vi "Camera AE V1.0.vi"(6 ".NET (Reference)":refnum<k24>, 7 "Camera Control In":T1 {"Frame Rate (fps)" scale=0.0..10.0; "Exposure Time (ms)" scale=0.0..10.0; "Pixel Clock (MHz)" scale=0.0..10.0}, 8 "Camera ID":i32, 9 "Action":T2) -> (0 "Error Out":errorcluster, 1 "Camera Control Out":T1 {"Frame Rate (fps)" scale=0.0..10.0; "Exposure Time (ms)" scale=0.0..10.0; "Pixel Clock (MHz)" scale=0.0..10.0}, 2 "Reference Out":refnum<k24>, 3 "Array":u8[][](array[numeric]))   [LabVIEW 2014]
uses:
  Controls/Standard Action for Camera Control.ctl
  C:/Program Files (x86)/National Instruments/LabVIEW 2014/instr.lib/IDS/ueye.NET/uEyeDotNet.dll
  Program Files (x86)/National Instruments/LabVIEW 2014/instr.lib/IDS/ueye.NET/uEyeDotNet.dll
  Controls/Camera Control.ctl
panel:
  out "Bits/Pixel":i32=8
  out "Width":i32=8
  out "Height":i32=8
  out "Serial Number 1":string
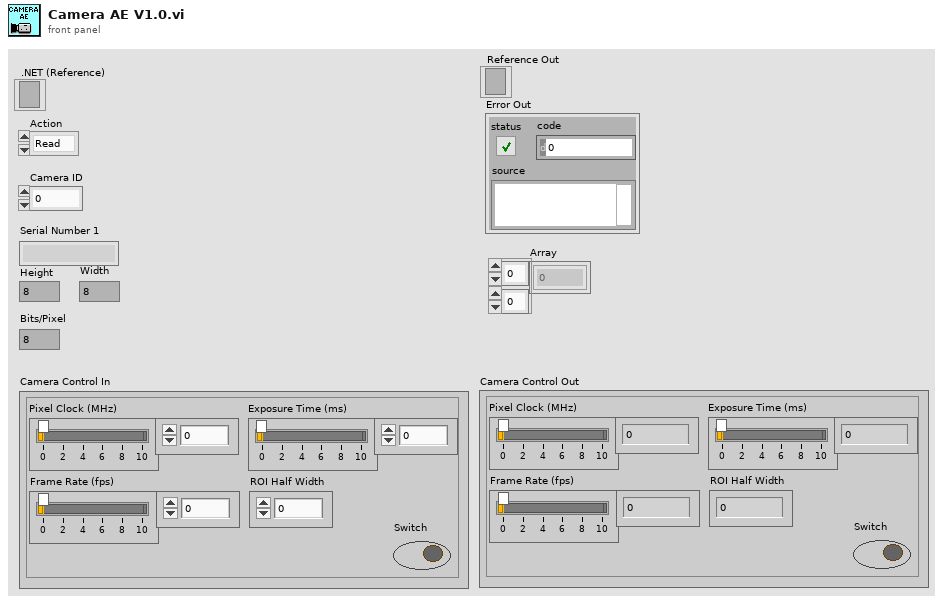
[diagram p1: front panel]
types:
  T1 = typedef "Camera Control.ctl" = cluster{"Pixel Clock (MHz)":i32, "Exposure Time (ms)":dbl, "Frame Rate (fps)":dbl, "ROI Half Width":i32, "Switch":bool}
  T2 = typedef "Standard Action for Camera Control.ctl" = enum16{"Read", "Setting", "Switch", "Initialization", "Exit"}
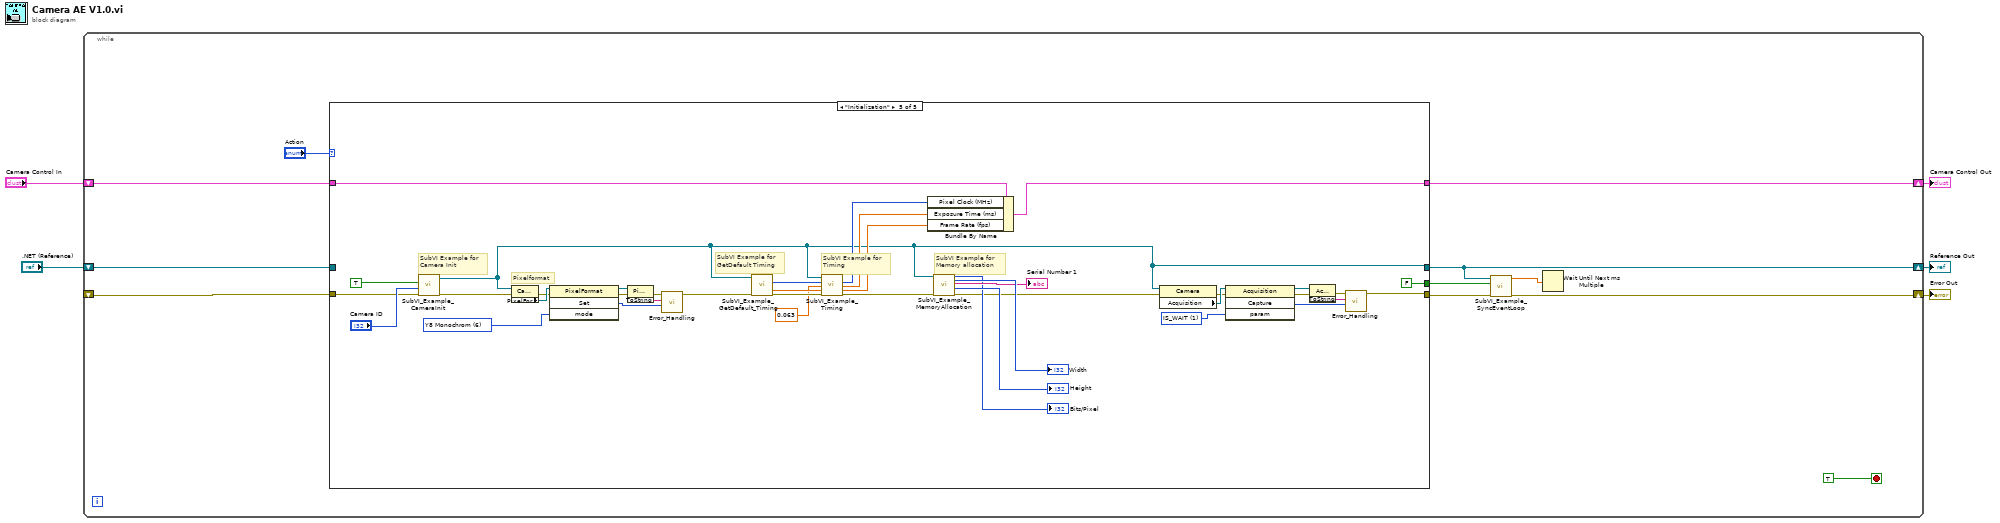
[diagram p0: block diagram]
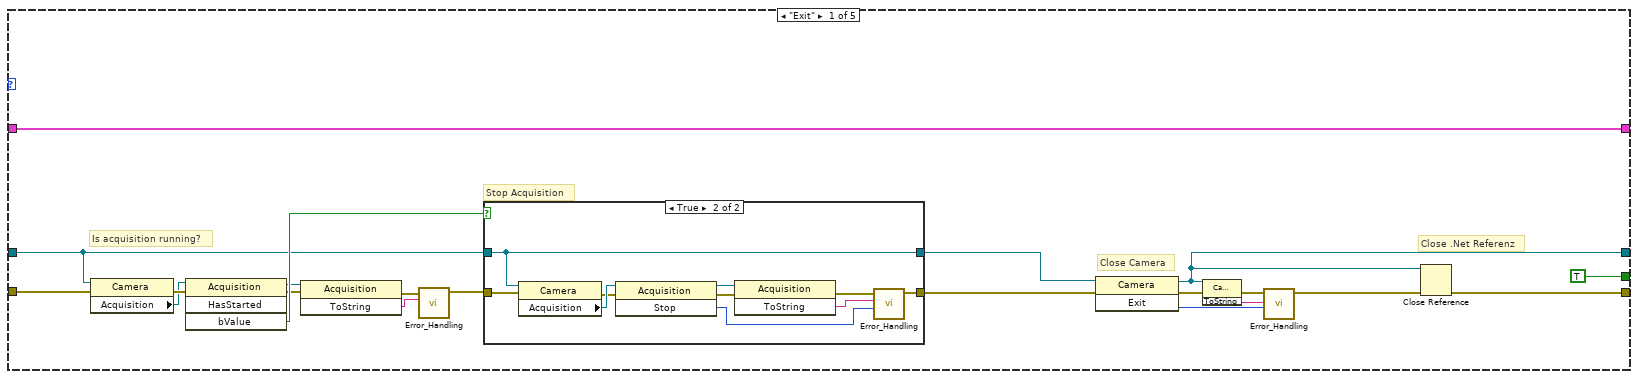
[diagram p2: hidden frame]
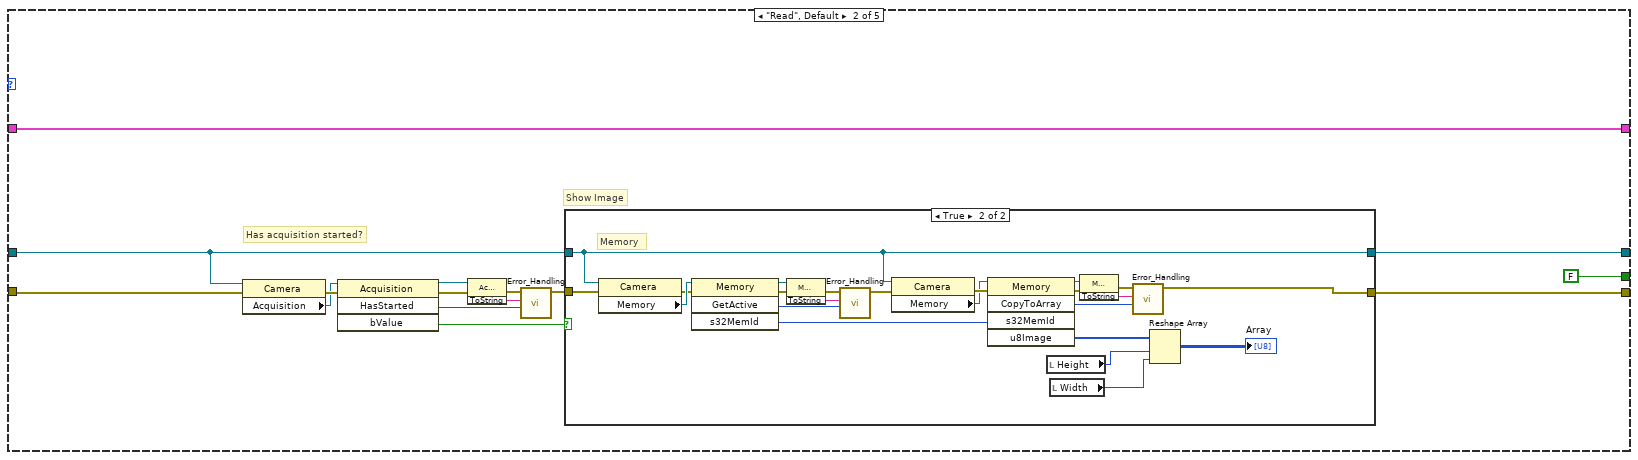
[diagram p4: hidden frame]
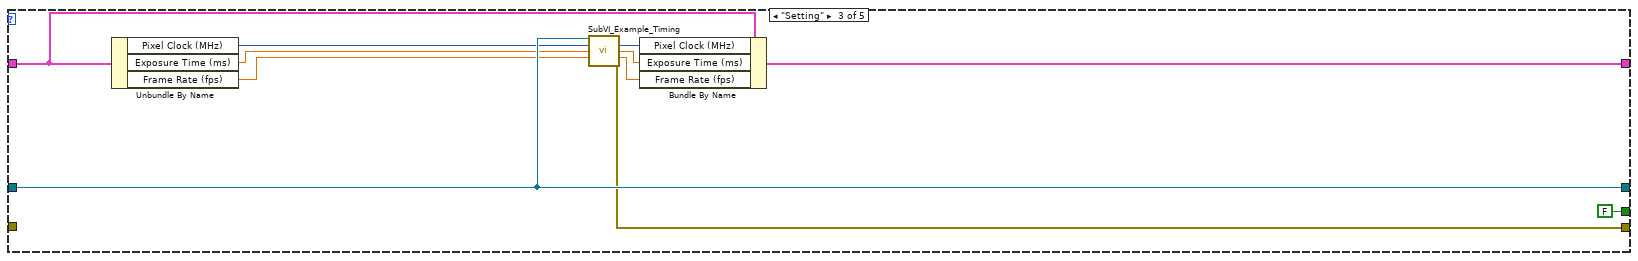
[diagram p6: hidden frame]
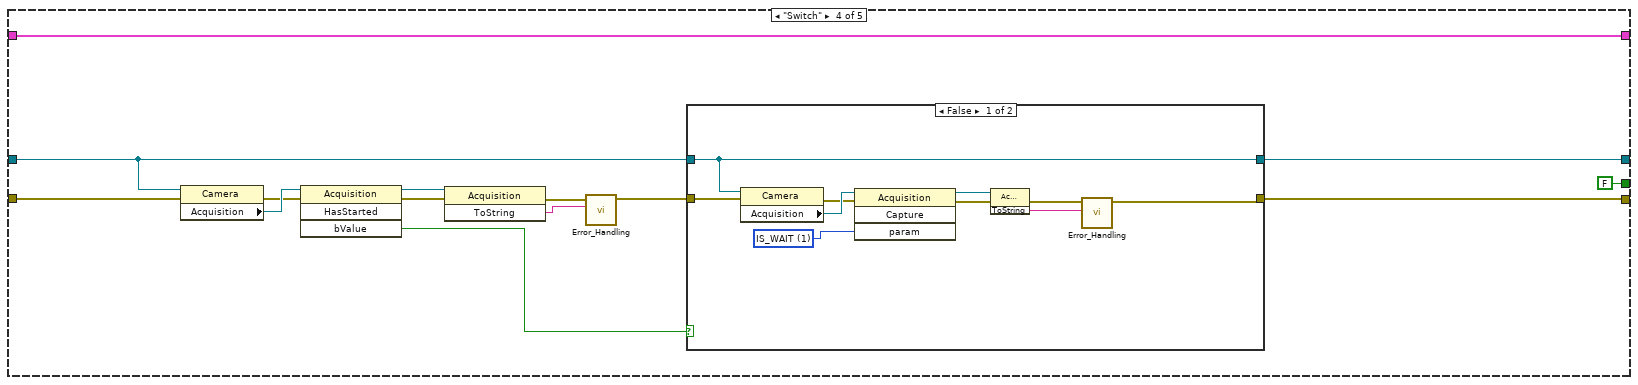
[diagram p7: hidden frame]
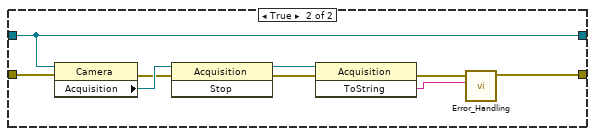
[diagram p8: hidden frame]
diagram:
  n1 = while {
    shift-right: [w12] -> w4
    shift-left: _ -> [w15]
    shift-right: [w13] -> w5
    shift-left: ".NET (Reference)" -> [w16]
    shift-right: [w7] -> w2
    shift-left: "Camera Control In" -> [w6]
    stop <- TRUE stop-if-true
    n2 = case shown="\"Initialization\"" "Action" {
      tunnel: w16 -> [w21 w53 w99 w101 _]
      tunnel: w15 -> [w22 w52 _ w114 w164]
      tunnel: [w31 w55 w99 w106 w136] -> w13
      tunnel: [w32 w54 w92 w103 w144] -> w14
      tunnel: [TRUE FALSE FALSE FALSE FALSE] -> w10
      tunnel: [w17 w50 w93 w111 w138] -> w7
      tunnel: w6 -> [w17 w50 w96 w111 w141]
      frame "Exit" {
        # "Close .Net Referenz"
        # "Is acquisition running?"
        # "Stop Acquisition"
        # "Close Camera"
        n3 = property class="Camera"(reference=w21, error in=w22) -> (error out=w30:errorcluster, "Acquisition"=w29:refnum<k24>)  [unwired: 1 out]
        n4 = invoke class="Acquisition" method="HasStarted"(reference=w29, error in=w30) -> (reference out=w23:refnum<k24>, error out=w26:errorcluster, "bValue"=w28:bool)  [unwired: 2 in, 1 out]
        n5 = invoke class="Acquisition" method="ToString"(reference=w23, error in=w26) -> (error out=w25:errorcluster, "ToString"=w24:string)  [unwired: 1 in, 1 out]
        n6 = call <instrlib>:"Error_Handling.vi"("Error String"=w24, "Error In"=w25) -> ("Error Out"=w27:errorcluster)  [unwired: 9 in]
        n7 = case shown="True" w28 {
          tunnel: [w39 w48] -> w19
          tunnel: w27 -> [w39 w49]
          tunnel: w21 -> [w38 w40]
          tunnel: [w38 w40] -> w20
          frame False {
          }
          frame True {
            n8 = property class="Camera"(reference=w40, error in=w49) -> (error out=w44:errorcluster, "Acquisition"=w45:refnum<k24>)  [unwired: 1 out]
            n9 = invoke class="Acquisition" method="Stop"(reference=w45, error in=w44) -> (reference out=w42:refnum<k24>, error out=w43:errorcluster, "Stop"=w41:i32)  [unwired: 1 in]
            n10 = invoke class="Acquisition" method="ToString"(reference=w42, error in=w43) -> (error out=w47:errorcluster, "ToString"=w46:string)  [unwired: 1 in, 1 out]
            n11 = call <instrlib>:"Error_Handling.vi"("Error Code"=w41, "Error String"=w46, "Error In"=w47) -> ("Error Out"=w48:errorcluster)  [unwired: 8 in]
          }
        }
        n12 = invoke class="Camera" method="Exit"(reference=w20, error in=w19) -> (reference out=w31:refnum<k24>, error out=w35:errorcluster, "Exit"=w34:i32)  [unwired: 1 in]
        n13 = invoke class="Camera" method="ToString"(reference=w31, error in=w35) -> (error out=w36:errorcluster, "ToString"=w37:string)  [unwired: 1 in, 1 out]
        n14 = call <instrlib>:"Error_Handling.vi"("Error Code"=w34, "Error String"=w37, "Error In"=w36) -> ("Error Out"=w33:errorcluster)  [unwired: 8 in]
        n15 = Close Reference ("Close Referenz")(reference=w31, error in (no error)=w33) -> (error out=w32:errorcluster)
      }
      frame "Read", Default {
        # "Has acquisition started?"
        # "Show Image"
        n16 = property class="Camera"(reference=w53, error in=w52) -> (error out=w64:errorcluster, "Acquisition"=w63:refnum<k24>)  [unwired: 1 out]
        n17 = invoke class="Acquisition" method="HasStarted"(reference=w63, error in=w64) -> (reference out=w59:refnum<k24>, error out=w58:errorcluster, "HasStarted"=w57:i32, "bValue"=w62:bool)  [unwired: 2 in]
        n18 = invoke class="Acquisition" method="ToString"(reference=w59, error in=w58) -> (error out=w61:errorcluster, "ToString"=w60:string)  [unwired: 1 in, 1 out]
        n19 = call <instrlib>:"Error_Handling.vi"("Error Code"=w57, "Error String"=w60, "Error In"=w61) -> ("Error Out"=w56:errorcluster)  [unwired: 8 in]
        n20 = case shown="True" w62 {
          tunnel: [w66 w71] -> w54
          tunnel: w56 -> [w66 w73]
          tunnel: w53 -> [w65 w72]
          tunnel: [w65 w72] -> w55
          frame False {
          }
          frame True {
            # "Memory"
            n21 = property class="Camera"(reference=w72, error in=w73) -> (error out=w75:errorcluster, "Memory"=w76:refnum<k24>)  [unwired: 1 out]
            n22 = invoke class="Memory" method="GetActive"(reference=w76, error in=w75) -> (reference out=w82:refnum<k24>, error out=w81:errorcluster, "GetActive"=w83:i32, "s32MemId"=w74:i32)  [unwired: 2 in]
            n23 = invoke class="Memory" method="ToString"(reference=w82, error in=w81) -> (error out=w79:errorcluster, "ToString"=w80:string)  [unwired: 1 in, 1 out]
            n24 = call <instrlib>:"Error_Handling.vi"("Error Code"=w83, "Error String"=w80, "Error In"=w79) -> ("Error Out"=w84:errorcluster)  [unwired: 8 in]
            n25 = property class="Camera"(reference=w72, error in=w84) -> (error out=w78:errorcluster, "Memory"=w77:refnum<k24>)  [unwired: 1 out]
            n26 = invoke class="Memory" method="CopyToArray"(reference=w77, error in=w78, "s32MemId"=w74) -> (reference out=w87:refnum<k24>, error out=w88:errorcluster, "CopyToArray"=w89:i32, "u8Image"=w70:u8[])  [unwired: 2 in, 1 out]
            n27 = local read "Height"() -> (w69:i32)
            n28 = local read "Width"() -> (w68:i32)
            n29 = invoke class="Memory" method="ToString"(reference=w87, error in=w88) -> (error out=w85:errorcluster, "ToString"=w86:string)  [unwired: 1 in, 1 out]
            n30 = call <instrlib>:"Error_Handling.vi"("Error Code"=w89, "Error String"=w86, "Error In"=w85) -> ("Error Out"=w71:errorcluster)  [unwired: 8 in]
            n31 = Reshape Array(w70, w69, w68) -> (→"Array":u8[][])
          }
        }
      }
      frame "Setting" {
        n32 = Unbundle By Name(w96) -> ("Pixel Clock (MHz)"=w98:i32, "Exposure Time (ms)"=w97:dbl, "Frame Rate (fps)"=w91:dbl)
        n33 = call <instrlib>:"SubVI_Example_Timing.vi"(".NET (Reference)"=w99, "Pixelclock"=w98, "Exposure time"=w97, "Framerate"=w91) -> ("Pixelclock"=w95:i32, "Exposure time"=w94:dbl, "Framerate"=w90:dbl, "Error Out"=w92:errorcluster)  [unwired: 8 in]
        n34 = Bundle By Name(cluster=w96, "Pixel Clock (MHz)"=w95, "Exposure Time (ms)"=w94, "Frame Rate (fps)"=w90) -> (w93:T1)
      }
      frame "Switch" {
        n35 = property class="Camera"(reference=w101, error in=w114) -> (error out=w112:errorcluster, "Acquisition"=w113:refnum<k24>)  [unwired: 1 out]
        n36 = invoke class="Acquisition" method="HasStarted"(reference=w113, error in=w112) -> (reference out=w110:refnum<k24>, error out=w109:errorcluster, "bValue"=w105:bool)  [unwired: 2 in, 1 out]
        n37 = invoke class="Acquisition" method="ToString"(reference=w110, error in=w109) -> (error out=w108:errorcluster, "ToString"=w107:string)  [unwired: 1 in, 1 out]
        n38 = call <instrlib>:"Error_Handling.vi"("Error String"=w107, "Error In"=w108) -> ("Error Out"=w104:errorcluster)  [unwired: 9 in]
        n39 = case shown="False" w105 {
          tunnel: w101 -> [w123 w132]
          tunnel: [w123 w132] -> w106
          tunnel: w104 -> [w124 w133]
          tunnel: [w115 w125] -> w103
          frame False {
            w121 = 1 items=["IS_DONT_WAIT", "IS_WAIT"] ("Wait")
            n40 = property class="Camera"(reference=w123, error in=w124) -> (error out=w120:errorcluster, "Acquisition"=w122:refnum<k24>)  [unwired: 1 out]
            n41 = invoke class="Acquisition" method="Capture"(reference=w122, error in=w120, "param"=w121) -> (reference out=w119:refnum<k24>, error out=w118:errorcluster)  [unwired: 1 in, 2 out]
            n42 = invoke class="Acquisition" method="ToString"(reference=w119, error in=w118) -> (error out=w117:errorcluster, "ToString"=w116:string)  [unwired: 1 in, 1 out]
            n43 = call <instrlib>:"Error_Handling.vi"("Error String"=w116, "Error In"=w117) -> ("Error Out"=w115:errorcluster)  [unwired: 9 in]
          }
          frame True {
            n44 = property class="Camera"(reference=w132, error in=w133) -> (error out=w130:errorcluster, "Acquisition"=w131:refnum<k24>)  [unwired: 1 out]
            n45 = invoke class="Acquisition" method="Stop"(reference=w131, error in=w130) -> (reference out=w129:refnum<k24>, error out=w128:errorcluster)  [unwired: 1 in, 1 out]
            n46 = invoke class="Acquisition" method="ToString"(reference=w129, error in=w128) -> (error out=w126:errorcluster, "ToString"=w127:string)  [unwired: 1 in, 1 out]
            n47 = call <instrlib>:"Error_Handling.vi"("Error String"=w127, "Error In"=w126) -> ("Error Out"=w125:errorcluster)  [unwired: 9 in]
          }
        }
      }
      frame "Initialization" {
        w145 = 1 items=["IS_DONT_WAIT", "IS_WAIT"] ("Wait")
        w172 = 6 items=["RGB 32"=0, "RGB 24"=1, "Y8 Monochrom"=6] ("Mode")
        # "SubVI Example for \nGetDefault Timing"
        # "SubVI Example for \nMemory allocation"
        # "SubVI Example for \nTiming"
        # "SubVI Example for \nCamera Init"
        # "Pixelformat"
        n48 = call <instrlib>:"SubVI_Example_CameraInit.vi"("Error In"=w164, "Camera ID"="Camera ID", "Init Camera Flag"=TRUE) -> ("Error Out"=w169:errorcluster, ".NET (Reference)"=w136:refnum<k24>)  [unwired: 7 in]
        n49 = property class="Camera"(reference=w136, error in=w169) -> (error out=w170:errorcluster, "PixelFormat"=w171:refnum<k24>)  [unwired: 1 out]
        n50 = invoke class="PixelFormat" method="Set"(reference=w171, error in=w170, "mode"=w172) -> (reference out=w167:refnum<k24>, error out=w162:errorcluster, "Set"=w166:i32)  [unwired: 1 in, 1 out]
        n51 = invoke class="PixelFormat" method="ToString"(reference=w167, error in=w162) -> (error out=w161:errorcluster, "ToString"=w168:string)  [unwired: 1 in, 1 out]
        n52 = call <instrlib>:"Error_Handling.vi"("Error Code"=w166, "Error String"=w168, "Error In"=w161) -> ("Error Out"=w155:errorcluster)  [unwired: 8 in]
        n53 = call <instrlib>:"SubVI_Example_GetDefault_Timing.vi"(".NET (Reference)"=w136, "Error In"=w155) -> ("Pixelclock"=w153:i32, "Framerate"=w154:dbl, "Error Out"=w143:errorcluster)  [unwired: 10 in, 1 out]
        n54 = call <instrlib>:"SubVI_Example_Timing.vi"(".NET (Reference)"=w136, "Pixelclock"=w153, "Exposure time"=0.063, "Framerate"=w154, "Error In"=w143) -> ("Pixelclock"=w140:i32, "Exposure time"=w139:dbl, "Framerate"=w137:dbl, "Error Out"=w160:errorcluster)  [unwired: 7 in]
        n55 = Bundle By Name(cluster=w141, "Pixel Clock (MHz)"=w140, "Exposure Time (ms)"=w139, "Frame Rate (fps)"=w137) -> (w138:T1)
        n56 = call <instrlib>:"SubVI_Example_MemoryAllocation.vi"(".NET (Reference)"=w136, "Error In"=w160) -> ("Bits/Pixel 2"=→"Bits/Pixel":i32, "Width"=→"Width":i32, "Serial Number"=→"Serial Number 1":string, "Height"=→"Height":i32, "Error Out"=w135:errorcluster)  [unwired: 13 in]
        n57 = property class="Camera"(reference=w136, error in=w135) -> (error out=w151:errorcluster, "Acquisition"=w152:refnum<k24>)  [unwired: 1 out]
        n58 = invoke class="Acquisition" method="Capture"(reference=w152, error in=w151, "param"=w145) -> (reference out=w147:refnum<k24>, error out=w148:errorcluster, "Capture"=w146:i32)  [unwired: 1 in, 1 out]
        n59 = invoke class="Acquisition" method="ToString"(reference=w147, error in=w148) -> (error out=w150:errorcluster, "ToString"=w149:string)  [unwired: 1 in, 1 out]
        n60 = call <instrlib>:"Error_Handling.vi"("Error Code"=w146, "Error String"=w149, "Error In"=w150) -> ("Error Out"=w144:errorcluster)  [unwired: 8 in]
      }
    }
    n61 = call <instrlib>:"SubVI_Example_SyncEventLoop.vi"("Error In"=w14, "use sync"=w10, ".NET (Reference)"=w13) -> ("Error Out"=w12:errorcluster, "Synchronize (ms)"=w11:dbl)  [unwired: 7 in]
    n62 = Wait Until Next ms Multiple(millisecond multiple=w11) -> ()  [unwired: 1 out]
  }
  "Reference Out" <- w5
  "Error Out" <- w4
  "Camera Control Out" <- w2
